vi "check constant multiple of polynomials (DBL).vi"(10 "Q(x)":dbl[](array[numeric]), 11 "P(x)":dbl[](array[numeric])) -> (3 "constant multiple?":bool)   [LabVIEW 2017, in "NI_AALPro.lvlib"]
uses:
  NI_AALPro.lvlib
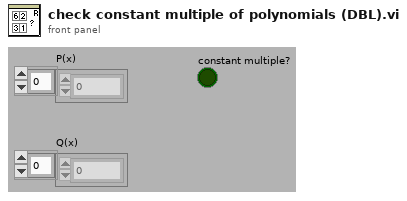
[diagram p1: front panel]
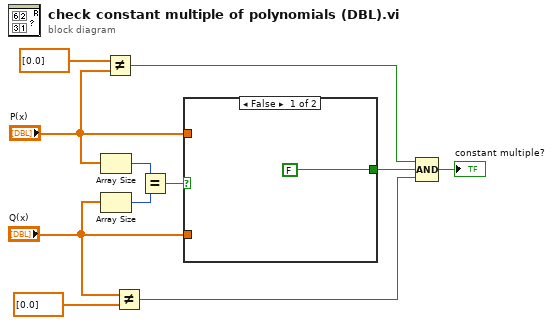
[diagram p0: block diagram]
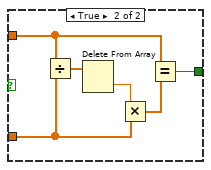
[diagram p2: hidden frame]
diagram:
  n1 = Array Size(array="P(x)") -> (size(s)=w11:i32)
  n2 = Array Size(array="Q(x)") -> (size(s)=w10:i32)
  n3 = Not Equal?(x=dbl[] [0.0] ("P(x)"), y="P(x)") -> (x != y?=w3:bool)
  n4 = Not Equal?(x="Q(x)", y=dbl[] [0.0] ("P(x)")) -> (x != y?=w2:bool)
  n5 = Equal?(x=w11, y=w10) -> (x = y?=w9:bool)
  n6 = case shown="False" w9 {
    tunnel: "Q(x)" -> [_ w18]
    tunnel: "P(x)" -> [_ w16]
    tunnel: [FALSE w17] -> w4
    frame False {
    }
    frame True {
      n7 = Divide(x=w16, y=w18) -> (x/y=w15:dbl[])
      n8 = Delete From Array(array=w15) -> (deleted portion=w14:dbl)  [unwired: 2 in, 1 out]
      n9 = Multiply(x=w14, y=w18) -> (x*y=w13:dbl[])
      n10 = Equal?(x=w16, y=w13) -> (x = y?=w17:bool)
    }
  }
  n11 = Compound Arithmetic op=AND(w3, w4, w2) -> (→"constant multiple?":bool)
